vi "Angle to hub.vi"(2 "Calculation Mode":enum16{"Theta Align", "Interp"}(ring), 3 "Robot Velocities In":T1={"X Velocity"=0.0, "Y Velocity"=-0.0, "Rotational \nVelocity"=0.0}, 4 "Time in flight":dbl, 5 "Using Limelight?":bool) -> (0 "Distance to hub":dbl, 1 "Angle to hub":dbl)   [LabVIEW 2025]
uses:
  swerve-template/Type Definitions/Data/Robot Velocities.ctl
  <vilib>/Rock Robotics/WPI/DriverStation/WPI_DriverStationAllianceInfo.ctl
  <vilib>/Rock Robotics/Network Tables/NT Read Numeric Array.vi
  Framework/Robot Global Data.vi
panel:
  out "Translation on Arc Pos":dbl
  out "Translation Against Arc Pos":dbl
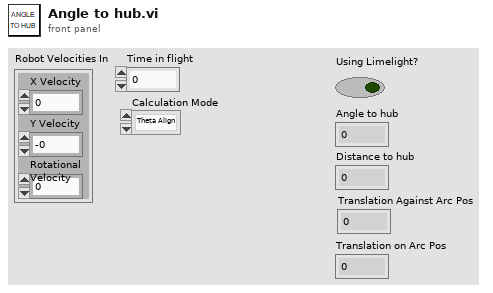
[diagram p1: front panel]
types:
  T1 = typedef "Robot Velocities.ctl" = cluster{"X Velocity":dbl, "Y Velocity":dbl, "Rotational \nVelocity":dbl}
  T2 = typedef "WPI_DriverStationAllianceInfo.ctl" = enum16{"Red", "Blue", "Invalid"}
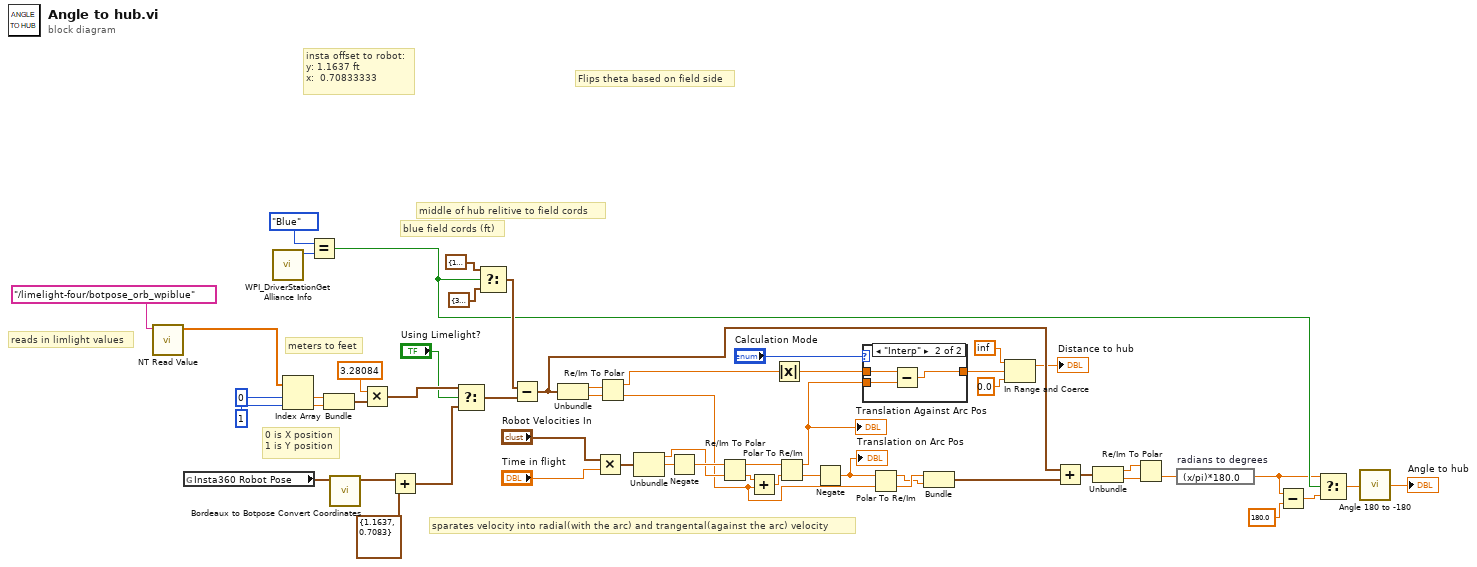
[diagram p0: block diagram]
diagram:
  # "insta offset to robot:\ny: 1.1637 ft\nx:  0.70833333"
  # "Flips theta based on field side"
  # "sparates velocity into radial(with the arc) and trangental(against the arc) velocity"
  # "blue field cords (ft)"
  # "middle of hub relitive to field cords"
  # "meters to feet"
  # "reads in limlight values"
  # "0 is X position\n1 is Y position"
  n1 = call-poly <vilib>:"NT Read Value.vi"("name"="/limelight-four/botpose_orb_wpiblue") -> ("value"=w46:dbl[])  [unwired: 8 in, 2 out]
  n2 = global read "Robot Global Data.vi" "Insta360 Robot Pose"() -> (w4:cluster{"X":dbl, "Y":dbl})
  n3 = call <vilib>:"WPI_DriverStationGet Alliance Info.vi"() -> ("Alliance"=w52:T2)  [unwired: 6 in, 5 out]
  n4 = Index Array(array=w46, index #1=0 ("index"), index #2=1 ("index")) -> (element #1=w48:dbl, element #2=w49:dbl)
  n5 = Equal?(x=WPI_DriverStationAllianceInfo."Blue", y=w52) -> (x = y?=w36:bool)
  n6 = Bundle("Numeric"=w48, "Numeric"=w49) -> (w47:cluster{"Numeric":dbl, "Numeric":dbl})  [unwired: 1 in]
  n7 = call "Bordeaux to Botpose Convert Coordinates.vi"("Pos In"=w4) -> ("Pos Out"=w3:cluster{dbl, dbl})  [unwired: 10 in]
  n8 = Multiply(x=3.28084, y=w47) -> (x*y=w7:cluster{"Numeric":dbl, "Numeric":dbl})
  n9 = Add(x=w3, y=cluster{dbl, dbl} {1.1637, 0.7083}) -> (x+y=w1:cluster{dbl, dbl})
  n10 = Select(t=w7, s="Using Limelight?", f=w1) -> (s? t:f=w6:cluster{"Numeric":dbl, "Numeric":dbl})
  n11 = Select(t=cluster{"Numeric":dbl, "Numeric":dbl} {"Numeric"=15.31, "Numeric"=13.19333} ("x"), s=w36, f=cluster{"Numeric":dbl, "Numeric":dbl} {"Numeric"=39.04667, "Numeric"=13.19333} ("x")) -> (s? t:f=w39:cluster{"Numeric":dbl, "Numeric":dbl})
  n12 = Subtract(x=w39, y=w6) -> (x-y=w25:cluster{"Numeric":dbl, "Numeric":dbl})
  n13 = Unbundle(w25) -> ("Numeric"=w35:dbl, "Numeric"=w34:dbl)
  n14 = Multiply(x="Robot Velocities In", y="Time in flight") -> (x*y=w40:T1)
  n15 = Re/Im To Polar(2:w34, 3:w35) -> (0:w26:dbl, 1:w55:dbl)
  n16 = Unbundle(w40) -> ("X Velocity"=w32:dbl, "Y Velocity"=w38:dbl)  [unwired: 1 out]
  n17 = Negate(x=w38) -> (-x=w33:dbl)
  n18 = Re/Im To Polar(2:w32, 3:w33) -> (0:w31:dbl, 1:w29:dbl)
  n19 = Add(x=w31, y=w26) -> (x+y=w30:dbl)
  n20 = Absolute Value(x=w55) -> (abs(x)=w27:dbl)
  n21 = Polar To Re/Im(2:w30, 3:w29) -> (0:w14:dbl, 1:w8:dbl)
  "Translation Against Arc Pos" <- w8
  n22 = Negate(x=w14) -> (-x=w9:dbl)
  "Translation on Arc Pos" <- w9
  n23 = case shown="\"Interp\"" "Calculation Mode" {
    tunnel: w27 -> [w57 w60]
    tunnel: w8 -> [_ w59]
    tunnel: [w57 w58] -> w18
    frame "Theta Align", Default {
    }
    frame "Interp" {
      n24 = Subtract(x=w60, y=w59) -> (x-y=w58:dbl)
    }
  }
  n25 = Polar To Re/Im(2:w26, 3:w9) -> (0:w11:dbl, 1:w10:dbl)
  n26 = Bundle(w11, w10) -> (w24:cluster{dbl, dbl})  [unwired: 1 in]
  n27 = In Range and Coerce(upper limit=inf, x=w18, lower limit=0.0) -> (coerced(x)=→"Distance to hub":dbl)  [unwired: 1 out]
  n28 = Add(x=w25, y=w24) -> (x+y=w23:cluster{dbl, dbl})
  n29 = Unbundle(w23) -> (w22:dbl, w21:dbl)
  n30 = Re/Im To Polar(2:w21, 3:w22) -> (0:w20:dbl)  [unwired: 1 out]
  n31 = expression code="(x/pi)*180.0" "radians to degrees"(w20) -> (w19:dbl)
  n32 = Subtract(x=w19, y=180.0 ("x")) -> (x-y=w54:dbl)
  n33 = Select(t=w19, s=w36, f=w54) -> (s? t:f=w13:dbl)
  n34 = call "Angle 180 to -180.vi"("Angle in"=w13) -> ("Angle out"=→"Angle to hub":dbl)
